vi "Rename DAQ Devices.vi"(0 "cDAQ Name":string="JL_SLB", 5 "DAQ Group":T1, 11 "Error In":errorcluster) -> (15 "Error Out":errorcluster)   [LabVIEW 2023]
uses:
  TypeDefs/Select DAQ Group.ctl
  <vilib>/nisyscfg/Initialize (Control).vi
  <vilib>/nisyscfg/Find Hardware.vi
  <vilib>/nisyscfg/Close (Filter).vi
  <vilib>/nisyscfg/Close (Hardware).vi
  <vilib>/nisyscfg/Close (System).vi
  <vilib>/nisyscfg/nisyscfg.lvlib
  <resource>/objmgr/nicontrollersysapi.rc
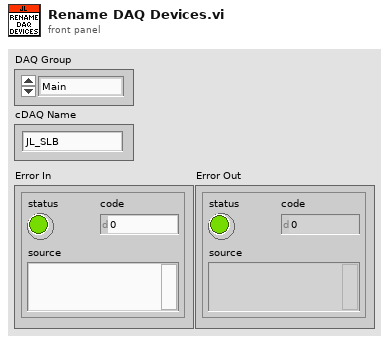
[diagram p1: front panel]
types:
  T1 = typedef "Select DAQ Group.ctl" = enum16{"Main", "Aux"}
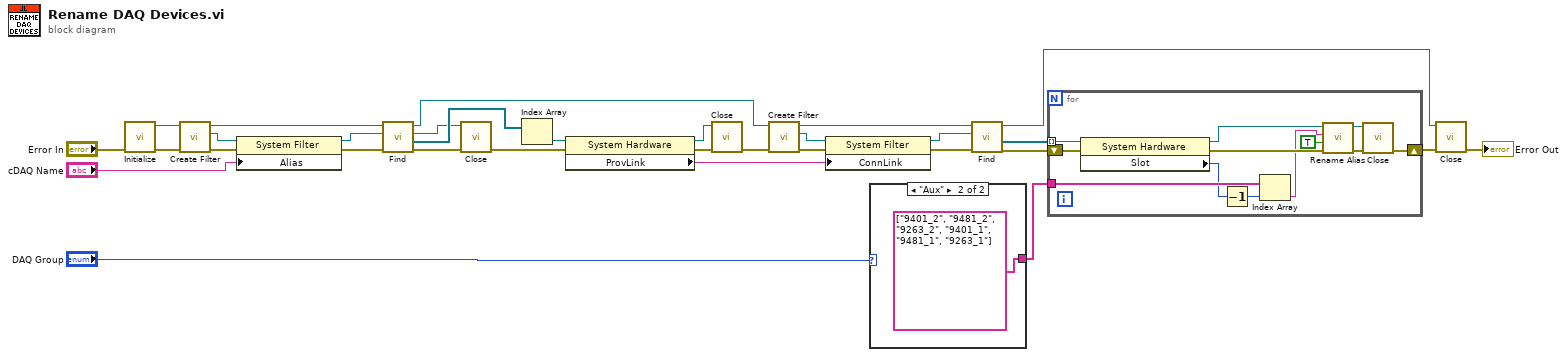
[diagram p0: block diagram]
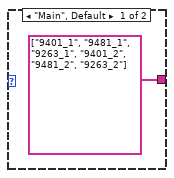
[diagram p2: hidden frame]
diagram:
  n1 = call-poly <vilib>:"Initialize.vi"("error in (no error)"="Error In") -> ("error out"=w30:errorcluster, "Session out"=w31:refnum<k21>)  [unwired: 8 in, 1 out]
  n2 = call <vilib>:"Create Filter.vi"("error in (no error)"=w30, "Session in"=w31) -> ("error out"=w28:errorcluster, "Filter out"=w29:refnum<k20>, "Session out"=w27:refnum<k21>)  [unwired: 7 in]
  n3 = property class="System Filter"(reference=w29, error in=w28, "Alias"="cDAQ Name") -> (reference out=w24:refnum<k20>, error out=w26:errorcluster)
  n4 = call-poly <vilib>:"Find.vi"("error in (no error)"=w26, "Filter in"=w24, "Session in"=w27) -> ("error out"=w13:errorcluster, "Resources out"=w21:refnum<k20>[], "Filter out"=w14:refnum<k20>, "Session out"=w11:refnum<k21>)  [unwired: 5 in]
  n5 = call-poly <vilib>:"Close.vi"("error in (no error)"=w13, "Filter in"=w14) -> ("error out"=w12:errorcluster)  [unwired: 9 in]
  n6 = Index Array(array=w21) -> (element=w20:refnum<k20>)  [unwired: 1 in]
  n7 = property class="System Hardware"(reference=w20, error in=w12) -> (reference out=w10:refnum<k20>, error out=w9:errorcluster, "ProvLink"=w7:string)
  n8 = call-poly <vilib>:"Close.vi"("error in (no error)"=w9, "Resource in"=w10) -> ("error out"=w8:errorcluster)  [unwired: 9 in]
  n9 = call <vilib>:"Create Filter.vi"("error in (no error)"=w8, "Session in"=w11) -> ("error out"=w16:errorcluster, "Filter out"=w15:refnum<k20>, "Session out"=w17:refnum<k21>)  [unwired: 7 in]
  n10 = property class="System Filter"(reference=w15, error in=w16, "ConnLink"=w7) -> (reference out=w19:refnum<k20>, error out=w18:errorcluster)
  n11 = case shown="\"Aux\"" "DAQ Group" {
    tunnel: [string[] ["9401_1", "9481_1", "9263_1", "9401_2", "9481_2", "9263_2"] string[] ["9401_2", "9481_2", "9263_2", "9401_1", "9481_1", "9263_1"]] -> w6
    frame "Main", Default {
    }
    frame "Aux" {
    }
  }
  n12 = call-poly <vilib>:"Find.vi"("error in (no error)"=w18, "Filter in"=w19, "Session in"=w17) -> ("error out"=w4:errorcluster, "Resources out"=w5:refnum<k20>[], "Session out"=w3:refnum<k21>)  [unwired: 5 in, 1 out]
  n13 = for {
    tunnel: w6 -> [w43]
    tunnel: w5 -> [w45] mode=indexing
    shift-right: [w39] -> w2
    shift-left: w4 -> [w44]
    n14 = property class="System Hardware"(reference=w45, error in=w44) -> (reference out=w37:refnum<k20>, error out=w40:errorcluster, "Slot"=w34:i32)
    n15 = Decrement(x=w34) -> (x-1=w35:i32)
    n16 = Index Array(array=w43, index=w35) -> (element=w38:string)
    n17 = call <vilib>:"Rename Alias.vi"("error in (no error)"=w40, "Overwrite Conflict (F)"=TRUE ("overwrite (F)"), "New Name"=w38, "Resource in"=w37) -> ("error out"=w41:errorcluster, "Resource out"=w36:refnum<k20>)  [unwired: 4 in, 2 out]
    n18 = call-poly <vilib>:"Close.vi"("error in (no error)"=w41, "Resource in"=w36) -> ("error out"=w39:errorcluster)  [unwired: 9 in]
  }
  n19 = call-poly <vilib>:"Close.vi"("error in (no error)"=w2, "Session in"=w3) -> ("error out"=→"Error Out":errorcluster)  [unwired: 9 in]
